vi "Get Tx Dataset.vi"(6 "Sequence Context In":refnum<k7>, 8 "error in":errorcluster, 10 "result_ready":bool, 11 "Fault FGVname":string="PLC Fault") -> (0 "error out":errorcluster, 3 "Tester Tx":T1)   [LabVIEW 2021, in "OPCUA.lvlib"]
uses:
  OPCUA.lvlib
  Controls/Tester Tx.ctl
  <vilib>/addons/TestStand/_TSUtility.llb/TestStand - Get Property Value (Number {Signed 32-bit Integer}).vi
  <vilib>/addons/TestStand/_TSUtility.llb/TestStand - Get Property Value (String).vi
  <vilib>/addons/TestStand/_TSUtility.llb/TestStand - Get Property Value (Number {Unsigned 32-bit Integer}).vi
  <vilib>/addons/TestStand/_TSUtility.llb/TestStand - Get Property Value (Numeric Array).vi
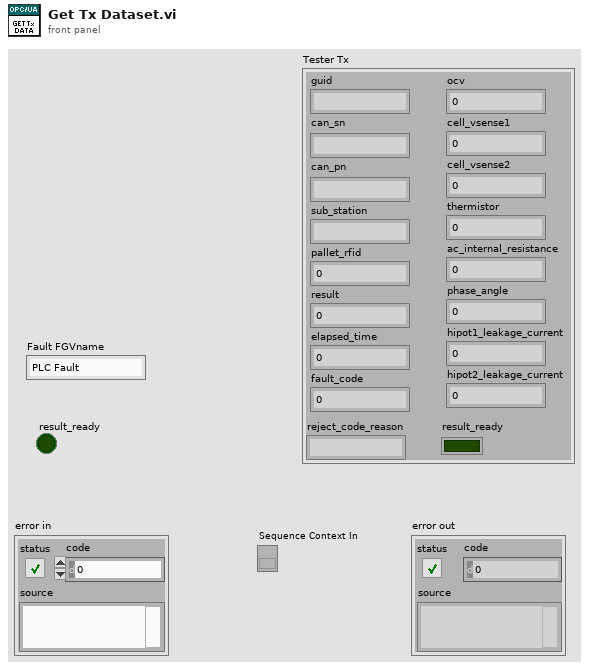
[diagram p1: front panel]
types:
  T1 = typedef "OPCUA.lvlib/Tester Tx.ctl" = cluster{"thermistor":dbl, "phase_angle":dbl, "pallet_rfid":dbl, "ocv":dbl, "cell_vsense1":dbl, "cell_vsense2":dbl, "hipot1_leakage_current":dbl, "hipot2_leakage_current":dbl, "guid":string, "can_sn":string, "can_pn":string, "ac_internal_resistance":dbl, "sub_station":string, "fault_code":i32, "elapsed_time":i32, "result":i32, "reject_code_reason":string, "result_ready":bool}
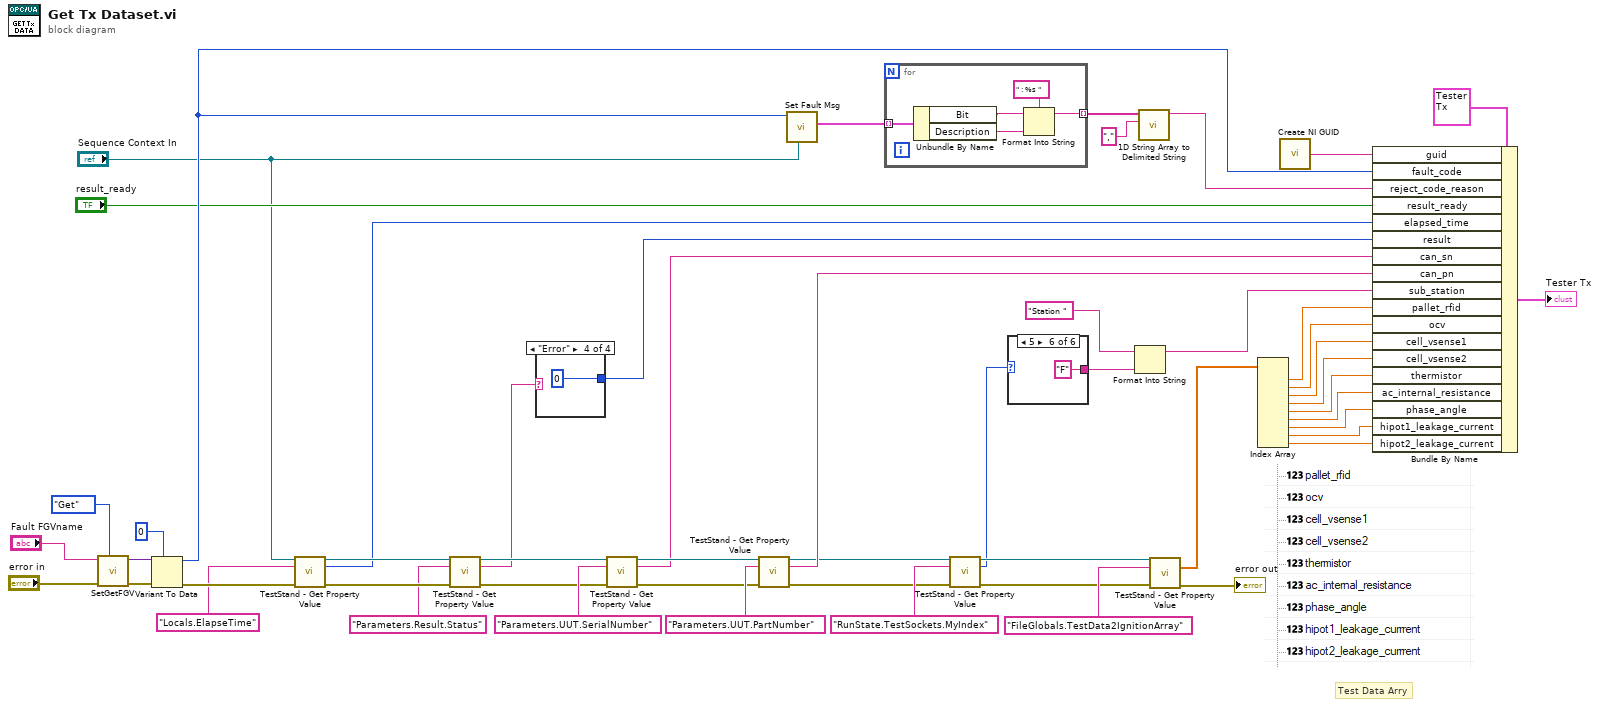
[diagram p0: block diagram]
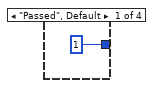
[diagram p2: hidden frame]
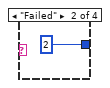
[diagram p3: hidden frame]
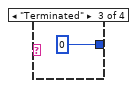
[diagram p4: hidden frame]
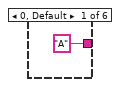
[diagram p5: hidden frame]
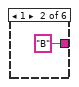
[diagram p6: hidden frame]
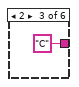
[diagram p7: hidden frame]
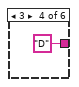
[diagram p8: hidden frame]
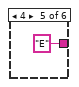
[diagram p9: hidden frame]
diagram:
  # "Test Data Arry"
  n1 = call "SetGetFGV.vi"("Method (Get)"=enum16{"Get", "Set"}."Get", "error in"="error in", "FGVname"="Fault FGVname") -> ("error out"=w23:errorcluster, "Data out"=w22:variant)  [unwired: 7 in]
  n2 = Variant To Data(error in=w23, type=u32 0 ("FaultCode"), Variant=w22) -> (data=w25:u32, error out=w8:errorcluster)
  n3 = call-poly <vilib>:"TestStand - Get Property Value.vi"("Sequence Context In"="Sequence Context In", "Lookup String"="Locals.ElapseTime", "error in (no error)"=w8) -> ("Sequence Context Out"=w9:refnum<k7>, "Value"=w3:i32, "error out"=w11:errorcluster)  [unwired: 10 in]
  n4 = call-poly <vilib>:"TestStand - Get Property Value.vi"("Sequence Context In"=w9, "Lookup String"="Parameters.Result.Status", "error in (no error)"=w11) -> ("Sequence Context Out"=w7:refnum<k7>, "Value"=w2:string, "error out"=w6:errorcluster)  [unwired: 10 in]
  n5 = case shown="\"Error\"" w2 {
    tunnel: [1 2 0 0] -> w1
    frame "Passed", Default {
    }
    frame "Failed" {
    }
    frame "Terminated" {
    }
    frame "Error" {
    }
  }
  n6 = call-poly <vilib>:"TestStand - Get Property Value.vi"("Sequence Context In"=w7, "Lookup String"="Parameters.UUT.SerialNumber", "error in (no error)"=w6) -> ("Sequence Context Out"=w52:refnum<k7>, "Value"=w48:string, "error out"=w50:errorcluster)  [unwired: 10 in]
  n7 = call-poly <vilib>:"TestStand - Get Property Value.vi"("Sequence Context In"=w52, "Lookup String"="Parameters.UUT.PartNumber", "error in (no error)"=w50) -> ("Sequence Context Out"=w28:refnum<k7>, "Value"=w47:string, "error out"=w45:errorcluster)  [unwired: 10 in]
  n8 = call "Set Fault Msg.vi"("Sequence Context"="Sequence Context In", "FaultCode"=w25) -> ("Fault codes"=w17:cluster{"Bit":string, "Description":string}[])  [unwired: 7 in, 2 out]
  n9 = for {
    tunnel: w17 -> [w60] mode=indexing
    tunnel: [w61] -> w15 mode=indexing
    n10 = Unbundle By Name(w60) -> ("Bit"=w58:string, "Description"=w59:string)
    n11 = Format Into String(format string=" : %s ", initial string=w58, w59) -> (resulting string=w61:string)  [unwired: 1 in, 1 out]
  }
  n12 = call-poly <vilib>:"TestStand - Get Property Value.vi"("Sequence Context In"=w28, "Lookup String"="RunState.TestSockets.MyIndex", "error in (no error)"=w45) -> ("Sequence Context Out"=w43:refnum<k7>, "Value"=w20:u32, "error out"=w41:errorcluster)  [unwired: 10 in]
  n13 = case shown="5" w20 {
    tunnel: ["A" ("format string") "B" ("format string") "C" ("format string") "D" ("format string") "E" ("format string") "F" ("format string")] -> w19
    frame 0, Default {
    }
    frame 1 {
    }
    frame 2 {
    }
    frame 3 {
    }
    frame 4 {
    }
    frame 5 {
    }
  }
  n14 = Format Into String(initial string="Station ", w19) -> (resulting string=w44:string)  [unwired: 2 in, 1 out]
  n15 = call <vilib>:"1D String Array to Delimited String.vi"("delimiter"=",", "string array"=w15) -> ("delimited string"=w14:string)  [unwired: 9 in]
  n16 = call-poly <vilib>:"TestStand - Get Property Value.vi"("Sequence Context In"=w43, "Lookup String"="FileGlobals.TestData2IgnitionArray", "error in (no error)"=w41) -> ("Value"=w40:dbl[], "error out"=→"error out":errorcluster)  [unwired: 10 in, 1 out]
  n17 = Index Array(array=w40) -> (element #1=w39:dbl, element #2=w38:dbl, element #3=w37:dbl, element #4=w36:dbl, element #5=w35:dbl, element #6=w34:dbl, element #7=w33:dbl, element #8=w32:dbl, element #9=w31:dbl)  [unwired: 9 in]
  n18 = call <vilib>:"Create NI GUID.vi"() -> ("NI GUID"=w29:string)
  n19 = Bundle By Name(cluster=T1 {"thermistor"=0.0, "phase_angle"=0.0, "pallet_rfid"=0.0, "ocv"=0.0, "cell_vsense1"=0.0, "cell_vsense2"=0.0, "hipot1_leakage_current"=0.0, "hipot2_leakage_current"=0.0, "guid"="", "can_sn"="", "can_pn"="", "ac_internal_resistance"=0.0, "sub_station"="", "fault_code"=0, "elapsed_time"=0, "result"=0, "reject_code_reason"="", "result_ready"=FALSE} ("Tester Tx"), "guid"=w29, "fault_code"=w25, "reject_code_reason"=w14, "result_ready"="result_ready", "elapsed_time"=w3, "result"=w1, "can_sn"=w48, "can_pn"=w47, "sub_station"=w44, "pallet_rfid"=w39, "ocv"=w38, "cell_vsense1"=w37, "cell_vsense2"=w36, "thermistor"=w35, "ac_internal_resistance"=w34, "phase_angle"=w33, "hipot1_leakage_current"=w32, "hipot2_leakage_current"=w31) -> (→"Tester Tx":T1)
